vi "loadClass.vi"(8 "error in (no error)":errorcluster, 10 "className":string, 11 "ClassLoader in":refnum<class "ClassLoader.lvclass">) -> (0 "error out":errorcluster, 2 "object out":refnum<class>, 3 "ClassLoader out":refnum<class "ClassLoader.lvclass">)   [LabVIEW 2020, in "JKI JSON Object Serialization.lvlib" / "OOP_Utility.lvlib" / "ClassLoader.lvclass"]
doc: "GCraftsman JSON Object Serialization Toolkit\nwww.GCraftsman.com\nCopyright (c) 2017, GCraftsman"
uses:
  ClassLoader.lvclass
  ClassLoader.lvclass/ClassLoader.ctl
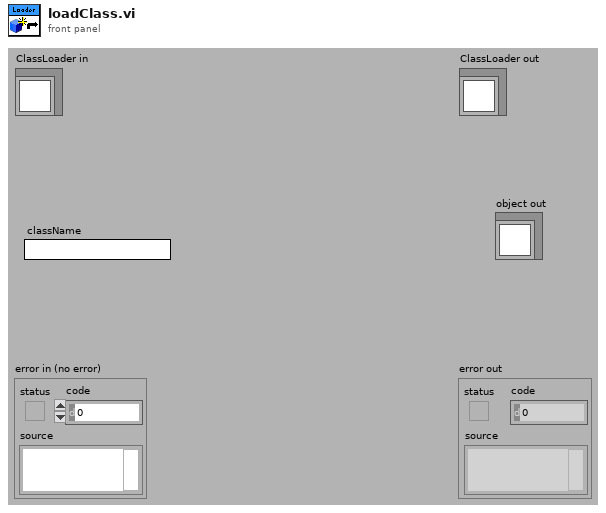
[diagram p1: front panel]
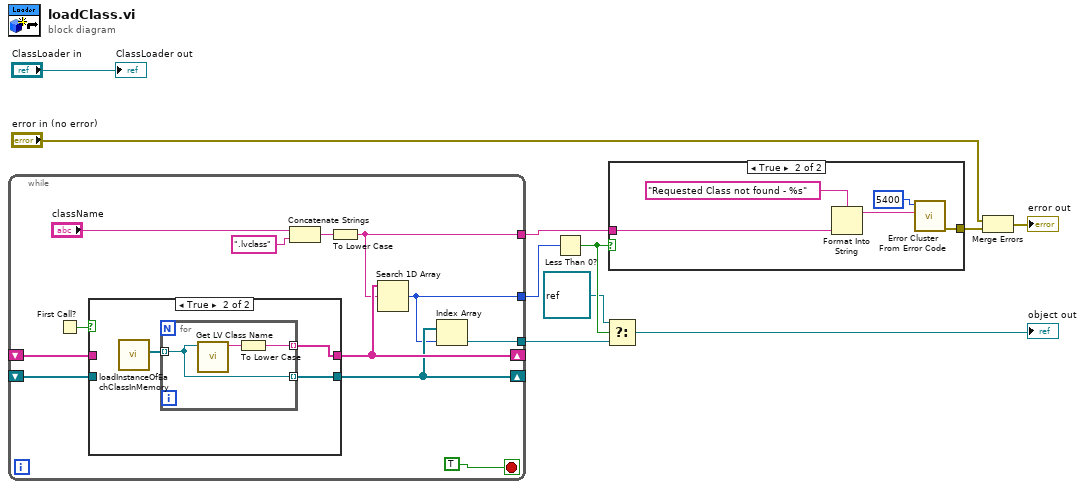
[diagram p0: block diagram]
diagram:
  n1 = while {
    shift-right: [w19] -> _
    shift-left: _ -> [w21]
    shift-right: [w17] -> _
    shift-left: _ -> [w20]
    tunnel: [w16] -> w1
    tunnel: [w15] -> w9
    tunnel: [w14] -> w8
    stop <- TRUE stop-if-true
    n2 = First Call?() -> (First Call?: T/F=w22:bool)
    n3 = case shown="True" w22 {
      tunnel: [w24 w27] -> w19
      tunnel: w21 -> [w24 _]
      tunnel: [w23 w26] -> w17
      tunnel: w20 -> [w23 _]
      frame False {
      }
      frame True {
        n4 = call "loadInstanceOfEachClassInMemory.vi"() -> ("all classes"=w25:refnum<class>[])  [unwired: 10 in, 1 out]
        n5 = for {
          tunnel: w25 -> [w29] mode=indexing
          tunnel: [w30] -> w27 mode=indexing
          tunnel: [w29] -> w26 mode=indexing
          n6 = call <vilib>:"Get LV Class Name.vi"("object"=w29) -> ("class name"=w28:string)  [unwired: 9 in, 1 out]
          n7 = To Lower Case(string=w28) -> (all lower case string=w30:string)
        }
      }
    }
    n8 = Concatenate Strings("className", ".lvclass" ("string")) -> (w11:string)
    n9 = To Lower Case(string=w11) -> (all lower case string=w14:string)
    n10 = Search 1D Array(1D array=w19, element=w14) -> (index of element=w15:i32)  [unwired: 1 in]
    n11 = Index Array(array=w17, index=w15) -> (element=w16:refnum<class>)
  }
  n12 = Less Than 0?(x=w9) -> (x < 0?=w5:bool)
  n13 = Select(t=refnum<class> refnum ("LabVIEW Object"), s=w5, f=w1) -> (s? t:f=→"object out":refnum<class>)
  n14 = case shown="True" w5 {
    tunnel: w8 -> [_ w34]
    tunnel: [_ w32] -> w2
    frame False {
    }
    frame True {
      n15 = Format Into String(format string="Requested Class not found - %s" ("message"), w34) -> (resulting string=w33:string)  [unwired: 2 in, 1 out]
      n16 = call <vilib>:"Error Cluster From Error Code.vi"("error message (\"\")"=w33, "error code (0)"=5400) -> ("error out"=w32:errorcluster)  [unwired: 7 in]
    }
  }
  n17 = Merge Errors("error in (no error)", w2) -> (→"error out":errorcluster)
  "ClassLoader out" <- "ClassLoader in"
